vi "BuildMenuRuntime.vi"(0 "XRef":T11, 1 "Point":T9, 2 "State In":T8) -> (14 "Menu Specification":T2, 15 "Fatal Error Out":T1)   [LabVIEW 2022 SP3, in "Flex Block.xnode"]
uses:
  Flex Block.xnode
  <vilib>/XNodeSupport/XNodeXNodeRef.ctl
  <vilib>/XNodeSupport/XNodePoint.ctl
  <vilib>/XNodeSupport/XNodeInt.ctl
  State.ctl
  <vilib>/XNodeSupport/XNodeMenuSpecs3.ctl
  <vilib>/XNodeSupport/XNodeMenuSpec3.ctl
  <vilib>/XNodeSupport/XNodeString.ctl
  <vilib>/XNodeSupport/XNodeBool.ctl
  <vilib>/XNodeSupport/XNodeStandardHelpInfo.ctl
  <vilib>/XNodeSupport/XNodePath.ctl
  <vilib>/XNodeSupport/XNodeErrorCluster.ctl
  <vilib>/XNodeSupport/NI_XNodeSupport.lvlib
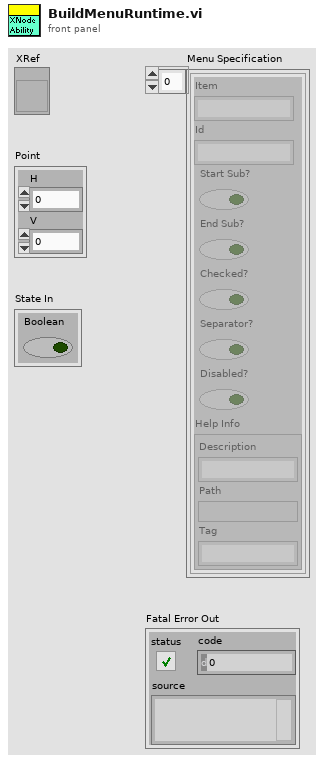
[diagram p1: front panel]
types:
  T1 = typedef "NI_XNodeSupport.lvlib/XNodeErrorCluster.ctl" = errorcluster
  T2 = typedef "NI_XNodeSupport.lvlib/XNodeMenuSpecs3.ctl" = T3[]
  T3 = typedef "NI_XNodeSupport.lvlib/XNodeMenuSpec3.ctl" = cluster{"Item":T4, "Id":T4, "Start Sub?":T5, "End Sub?":T5, "Checked?":T5, "Separator?":T5, "Disabled?":T5, "Help Info":T6}
  T4 = typedef "NI_XNodeSupport.lvlib/XNodeString.ctl" = string
  T5 = typedef "NI_XNodeSupport.lvlib/XNodeBool.ctl" = bool
  T6 = typedef "NI_XNodeSupport.lvlib/XNodeStandardHelpInfo.ctl" = cluster{"Description":T4, "Path":T7, "Tag":T4}
  T7 = typedef "NI_XNodeSupport.lvlib/XNodePath.ctl" = path
  T8 = typedef "Flex Block.xnode/State.ctl" = cluster{"Boolean":bool}
  T9 = typedef "NI_XNodeSupport.lvlib/XNodePoint.ctl" = cluster{"H":T10, "V":T10}
  T10 = typedef "NI_XNodeSupport.lvlib/XNodeInt.ctl" = i32
  T11 = typedef "NI_XNodeSupport.lvlib/XNodeXNodeRef.ctl" = refnum<vi>
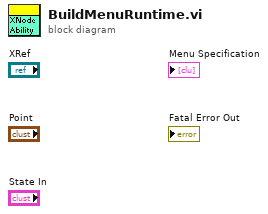
[diagram p0: block diagram]
diagram:
